vi "Remove Array Outliers.vi"(8 "Error In":errorcluster, 9 "Upper & Lower Percentile (100, 0)":dbl[](array[numeric])=[1.0, 0.0], 11 "Array in":dbl[](array[numeric])) -> (0 "Error Out":errorcluster, 1 "# Rejected Elements":i32, 3 "Array out":dbl[](array[numeric]))   [LabVIEW 2021, in "Arrays.lvlib"]
uses:
  Arrays.lvlib
  <vilib>/Utility/error.llb/Error Cluster From Error Code.vi
  <vilib>/Comparison/Less/Less Functor/Less Functor.lvclass
  <vilib>/ErrorRing/Error Ring.xnode
  <vilib>/gmath/NI_Gmath.lvlib
  Error/Error.lvlib
  <vilib>/gmath/statdist.llb/st_Percentiles (array).vi
panel:
  # "see the License on the block diagram (Ctrl+E or Window:Show Block Diagram)"
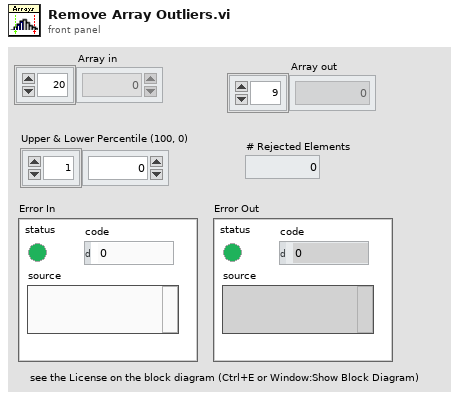
[diagram p1: front panel]
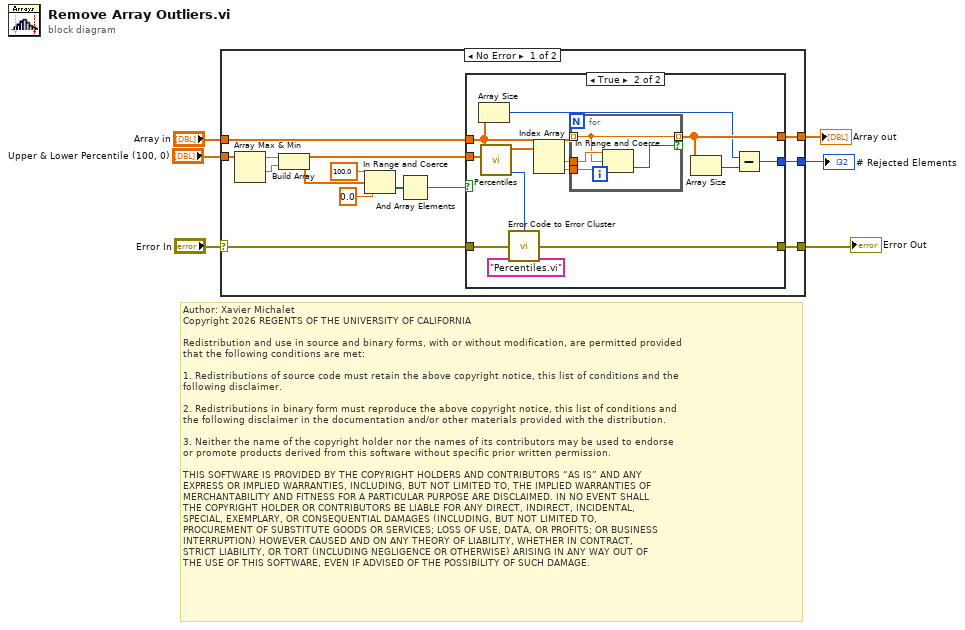
[diagram p0: block diagram]
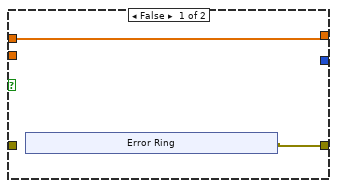
[diagram p2: hidden frame]
diagram:
  # "Author: Xavier Michalet\nCopyright 2026 REGENTS OF THE UNIVERSITY OF CALIFORNIA\n\nRedistribution and use in source and binary forms, with or without modification, are permitted provided\nthat the following conditions are met:\n\n1. Redistributions of source code must retain the above copyright notice, this list of conditions and the\nfollowing disclaimer.\n\n2. Redistributions in binary form must reproduce the above copyright notice, this list of conditions and\nthe following disclaimer in the documentation and/or other materials provided with the distribution.\n\n3. Neither the name of the copyright holder nor the names of its contributors may be used to endorse \nor promote products derived from this software without specific prior written permission.\n\nTHIS SOFTWARE IS PROVIDED BY THE COPYRIGHT HOLDERS AND CONTRIBUTORS “AS IS” AND ANY \nEXPRESS OR IMPLIED WARRANTIES, INCLUDING, BUT NOT LIMITED TO, THE IMPLIED WARRANTIES OF\nMERCHANTABILITY AND FITNESS FOR A PARTICULAR PURPOSE ARE DISCLAIMED. IN NO EVENT SHALL\nTHE COPYRIGHT HOLDER OR CONTRIBUTORS BE LIABLE FOR ANY DIRECT, INDIRECT, INCIDENTAL, \nSPECIAL, EXEMPLARY, OR CONSEQUENTIAL DAMAGES (INCLUDING, BUT NOT LIMITED TO, \nPROCUREMENT OF SUBSTITUTE GOODS OR SERVICES; LOSS OF USE, DATA, OR PROFITS; OR BUSINESS\nINTERRUPTION) HOWEVER CAUSED AND ON ANY THEORY OF LIABILITY, WHETHER IN CONTRACT, \nSTRICT LIABILITY, OR TORT (INCLUDING NEGLIGENCE OR OTHERWISE) ARISING IN ANY WAY OUT OF\nTHE USE OF THIS SOFTWARE, EVEN IF ADVISED OF THE POSSIBILITY OF SUCH DAMAGE."
  n1 = case shown="No Error" "Error In" {
    selector: "Error In" -> [w14 w43]
    tunnel: [w19 w44] -> w6
    tunnel: "Array in" -> [w18 w44]
    tunnel: "Upper & Lower Percentile (100, 0)" -> [w11 _]
    tunnel: [w13 w43] -> w2
    tunnel: [w12 _] -> w1
    frame No Error {
      n2 = Array Max & Min(array=w11) -> (max value=w10:dbl, min value=w9:dbl)  [unwired: 2 out]
      n3 = Build Array(w10, w9) -> (w8:dbl[])
      n4 = In Range and Coerce(upper limit=100.0, x=w8, lower limit=0.0) -> (In Range?=w15:bool[])  [unwired: 1 out]
      n5 = And Array Elements(Boolean array=w15) -> (logical AND=w7:bool)
      n6 = case shown="True" w7 {
        tunnel: [w21 w31] -> w19
        tunnel: w18 -> [w21 w30]
        tunnel: w8 -> [_ w35]
        tunnel: w14 -> [_ w34]
        tunnel: [w20 w32] -> w13
        tunnel: [_ w27] -> w12
        frame False {
          n7 = xnode "Error Ring"() -> ("error out"=w20:errorcluster)
        }
        frame True {
          n8 = Array Size(array=w30) -> (size(s)=w28:i32)
          n9 = call-poly <vilib>:"Percentiles.vi"("p array"=w35, "x array"=w30) -> ("error"=w33:i32, "percentiles"=w36:dbl[])  [unwired: 8 in]
          n10 = call "Error Code to Error Cluster.vi"("Error Code"=w33, "Error Source"="Percentiles.vi", "Error In"=w34) -> ("Error Out"=w32:errorcluster)  [unwired: 12 in]
          n11 = Index Array(array=w36) -> (element #1=w37:dbl, element #2=w38:dbl)  [unwired: 2 in]
          n12 = for {
            tunnel: w30 -> [w40] mode=indexing
            tunnel: w37 -> [w42]
            tunnel: w38 -> [w41]
            tunnel: [w40] -> w31 mode=indexing if=w39
            n13 = In Range and Coerce(upper limit=w42, x=w40, lower limit=w41) -> (In Range?=w39:bool)  [unwired: 1 out]
          }
          n14 = Array Size(array=w31) -> (size(s)=w29:i32)
          n15 = Subtract(x=w28, y=w29) -> (x-y=w27:i32)
        }
      }
    }
    frame Error {
    }
  }
  "Array out" <- w6
  "Error Out" <- w2
  "# Rejected Elements" <- w1
